vi "Plot refnum Write.vi"(4 "error in (no error)":errorcluster, 5 "Value":refnum<vi>, 6 "Container State":T2, 7 "Display State In":T1) -> (0 "error out":errorcluster, 3 "Display State Out":T1)   [LabVIEW 2020, in "KLegend.xctl"]
uses:
  KLegend.xctl
  <vilib>/_xctls/Container State.ctl
  State.vi
  <vilib>/_xctls/XControlSupport.lvlib
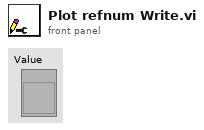
[diagram p1: front panel]
types:
  T1 = typedef "KLegend.xctl/State.vi" = cluster{"Plot":refnum<vi>, "Vals":dbl[], "fmt":string, "cmd":string, "max rows":i32}
  T2 = typedef "XControlSupport.lvlib/Container State.ctl" = cluster{"Indicator?":bool, "Run Mode?":bool, " Refnum":refnum<vi>}
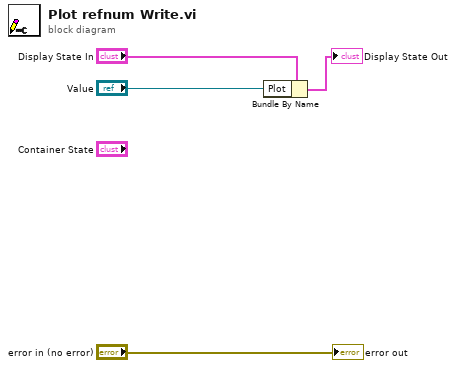
[diagram p0: block diagram]
diagram:
  n1 = Bundle By Name(cluster="Display State In", "Plot"="Value") -> (→"Display State Out":T1)
  "error out" <- "error in (no error)"
